vi "Read Density.vi"(8 "error in (no error)":errorcluster, 11 "Moving Ripple Noise in":refnum<class "Moving Ripple Noise.lvclass">) -> (0 "error out":errorcluster, 2 "Density":dbl, 3 "Moving Ripple Noise out":refnum<class "Moving Ripple Noise.lvclass">)   [LabVIEW 2020, in "Moving Ripple Noise.lvclass"]
uses:
  Moving Ripple Noise.lvclass
  Moving Ripple Noise.lvclass/Moving Ripple Noise.ctl
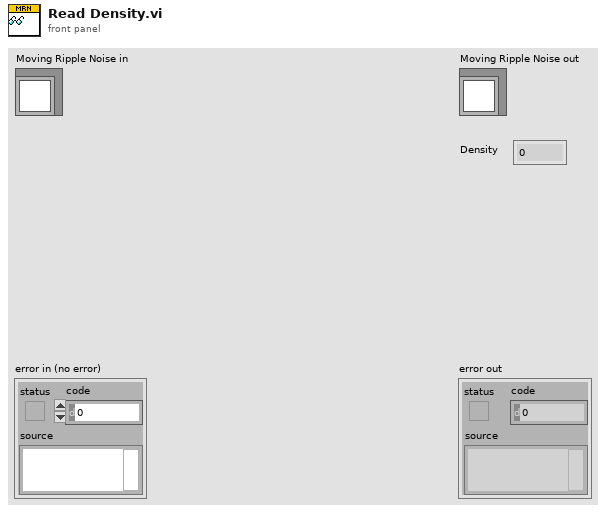
[diagram p1: front panel]
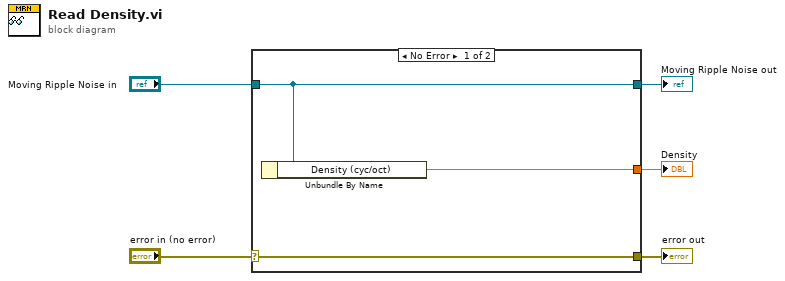
[diagram p0: block diagram]
diagram:
  n1 = case shown="No Error" "error in (no error)" {
    selector: "error in (no error)" -> [w8 w9]
    tunnel: [w8 w9] -> w4
    tunnel: [w7 w10] -> w2
    tunnel: "Moving Ripple Noise in" -> [w7 w10]
    tunnel: [w6 _] -> w1
    frame No Error {
      n2 = Unbundle By Name(w7) -> ("Density (cyc/oct)"=w6:dbl)
    }
    frame Error {
    }
  }
  "error out" <- w4
  "Moving Ripple Noise out" <- w2
  "Density" <- w1
